vi ".Launch Vaisala.vi"(8 "Error In":errorcluster, 11 "TEC Controller in":refnum<class "TEC Controller.lvclass">) -> (0 "error out":errorcluster, 2 "ID":string, 3 "TEC Controller out":refnum<class "TEC Controller.lvclass">)   [LabVIEW 2014, in "Humidifier Test Lib.lvlib" / "TEC Controller.lvclass"]
uses:
  TEC Controller.lvclass
  reusable/Session APIs/Session Log/System Log.lvclass
  reusable/Session APIs/File Access/Config Data/Config Data.lvclass
  reusable/DAQ Device/Device/Device.lvclass
  Messages for Controller/Update Data MSG/Update Humidifier Controller MSG.lvclass
  Devices/Vaisala Probe/Vaisala.lvclass
  TEC Controller.lvclass/TEC Controller.ctl
  reusable/Session APIs/File Access/Config Data/Config Data.lvclass/Config Data.ctl
  reusable/Session APIs/Session Log/System Log.lvclass/System Log.ctl
  Devices/Configurable Device/Configurable Device.lvclass/Configurable Device.ctl
  reusable/DAQ Device/Device/Generic Data Update Data MSG/Generic Update Data Message.lvclass/Generic Update Data Message.ctl
  reusable/DAQ Device/Device/Device.lvclass/Device.ctl
  SuperActor/Ex Nested.lvclass/Ex Nested.ctl
  reusable/Session APIs/File Access/Config Data/Accessors/Write Cfg Path.vi
  reusable/Session APIs/Session Log/Accessors/Write Main Path.vi
  Devices/Configurable Device/Write Log Session.vi
  Devices/Configurable Device/Write Handle.vi
  Devices/Configurable Device/Write ID.vi
  reusable/DAQ Device/Device/Generic Data Update Data MSG/Write ID.vi
  reusable/DAQ Device/Device/Write Update Period.vi
  reusable/DAQ Device/Device/Write Configurable Device.vi
  reusable/DAQ Device/Device/Write Update MSG.vi
  SuperActor/Write ID.vi
  reusable/Session APIs/File Access/Config Data/Read Array/Read String Array.vi
  <userlib>/_Session Fwk/Session - Root.lvclass
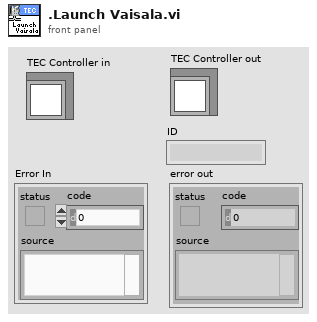
[diagram p1: front panel]
types:
  T1 = typedef "Session - Root.lvclass/Session Handle.ctl" = refnum<data-value>
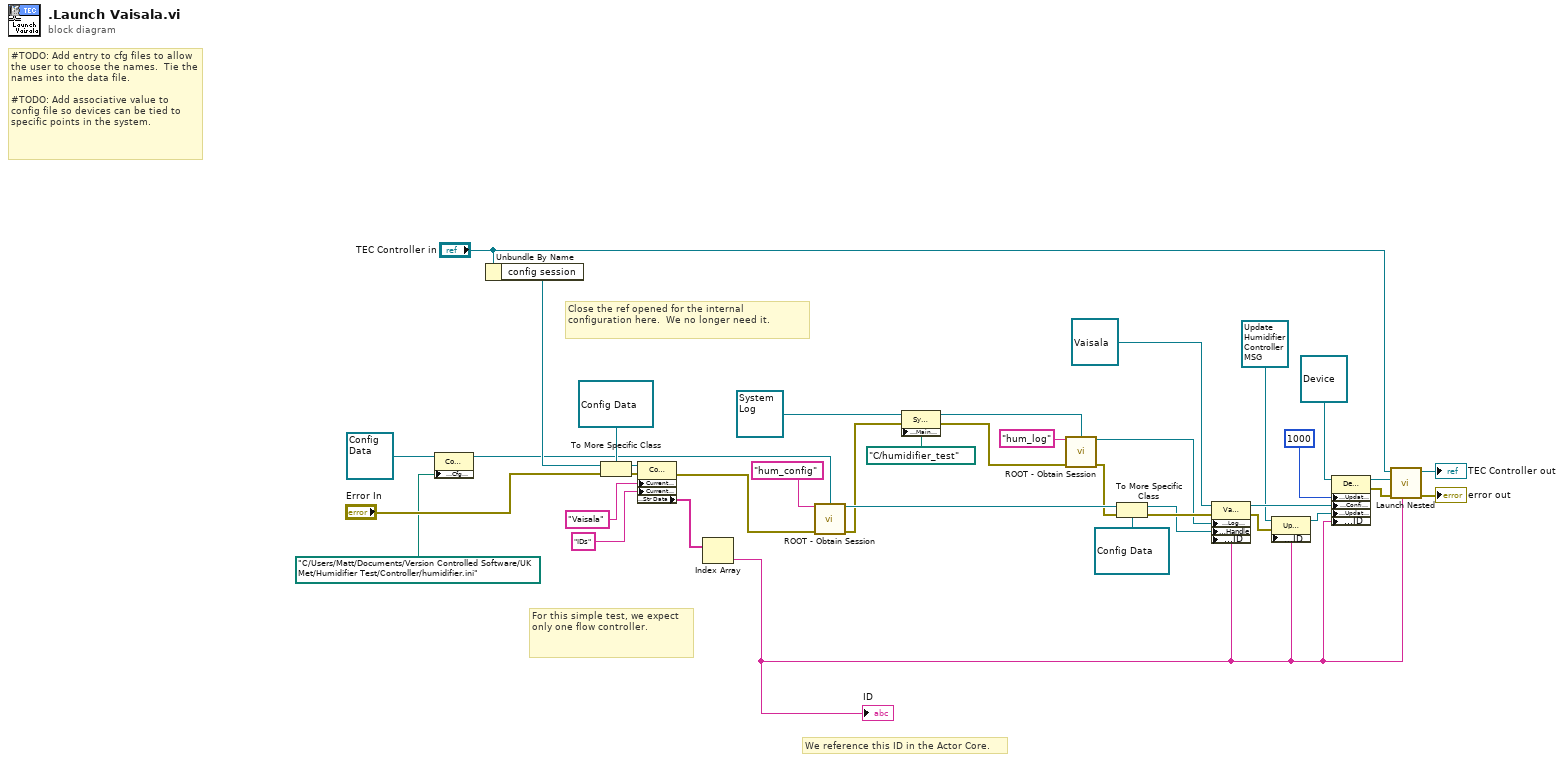
[diagram p0: block diagram]
diagram:
  # "We reference this ID in the Actor Core."
  # "Close the ref opened for the internal configuration here.  We no longer need it."
  # "For this simple test, we expect only one flow controller."
  # "#TODO: Add entry to cfg files to allow the user to choose the names.  Tie the names into the data file.\n\n#TODO: Add associative value to config file so devices can be tied to specific points in the system."
  n1 = property class="Config Data"(reference=refnum<class "Config Data.lvclass"> refnum ("Config Data"), "Accessors:Cfg Path"=path "C:/Users/Matt/Documents/Version Controlled Software/UK Met/Humidifier Test/Controller/humidifier.ini" ("Main Path")) -> (reference out=w2:refnum<class "Config Data.lvclass">)  [unwired: 1 in, 1 out]
  n2 = Unbundle By Name("TEC Controller in") -> ("config session"=w7:T1)
  n3 = To More Specific Class(target class=refnum<data-value> refnum ("Session Handle"), reference=w7, error in="Error In") -> (specific class reference=w36:refnum<data-value>, error out=w15:errorcluster)
  n4 = property class="Config Data"(reference=w36, error in=w15, "Current Section"="Vaisala", "Current Key"="IDs") -> (error out=w30:errorcluster, "Read Array Data:Str Data"=w33:string[])  [unwired: 1 out]
  n5 = Index Array(array=w33) -> (element=w16:string)  [unwired: 1 in]
  "ID" <- w16
  n6 = call <userlib>:"ROOT - Obtain Session.vi"("Session Name ()"="hum_config", "OBJ - Session"=w2, "error in (no error)"=w30) -> ("Session Handle"=w29:T1, "error out"=w13:errorcluster)  [unwired: 10 in, 1 out]
  n7 = property class="Sys Log"(reference=refnum<class "System Log.lvclass"> refnum ("Sys Log"), error in=w13, "Accessors:Main Path"=path "C:/humidifier_test" ("Main Path")) -> (reference out=w31:refnum<class "System Log.lvclass">, error out=w14:errorcluster)
  n8 = call <userlib>:"ROOT - Obtain Session.vi"("Session Name ()"="hum_log", "OBJ - Session"=w31, "error in (no error)"=w14) -> ("Session Handle"=w11:T1, "error out"=w12:errorcluster)  [unwired: 10 in, 1 out]
  n9 = To More Specific Class(target class=refnum<data-value> refnum ("Session Handle"), reference=w29, error in=w12) -> (specific class reference=w10:refnum<data-value>, error out=w27:errorcluster)
  n10 = property class="Vaisala"(reference=refnum<class "Vaisala.lvclass"> refnum ("Vaisala Library.lvlib:Vaisala"), error in=w27, "Accessors:Log Session"=w11, "Accessors:Handle"=w10, "Accessors:ID"=w16) -> (reference out=w38:refnum<class "Vaisala.lvclass">, error out=w9:errorcluster)
  n11 = property class="Update Humidifier Controller"(reference=refnum<class "Update Humidifier Controller MSG.lvclass"> refnum ("Humidifier Test Lib.lvlib:Update Humidifier Controller"), error in=w9, "Accessors:ID"=w16) -> (reference out=w24:refnum<class "Update Humidifier Controller MSG.lvclass">)  [unwired: 1 out]
  n12 = property class="Device"(reference=refnum<class "Device.lvclass"> refnum ("DAQ Device.lvlib:Device"), "Accessors:Update Period"=1000 ("Update Period"), "Accessors:Configurable Device"=w38, "Accessors:Update MSG"=w24, "Accessors:ID"=w16) -> (reference out=w23:refnum<class "Device.lvclass">, error out=w22:errorcluster)  [unwired: 1 in]
  n13 = call "Launch Nested.vi"("ID"=w16, "error in (no error)"=w22, "Nested Actor"=w23, "TEC Controller in"="TEC Controller in") -> ("error out"=→"error out":errorcluster, "TEC Controller out"=→"TEC Controller out":refnum<class "TEC Controller.lvclass">)  [unwired: 6 in]
